vi "updateTimestamp.vi"(8 "error in (no error)":errorcluster, 10 "Timestamp":dbl, 11 "Timestamp in":refnum<class "Timestamp.lvclass">) -> (0 "error out":errorcluster, 3 "Timestamp out":refnum<class "Timestamp.lvclass">)   [LabVIEW 2016, in "RTTimestamp.lvlib" / "Timestamp.lvclass"]
uses:
  Timestamp.lvclass
  Timestamp.lvclass/Timestamp.ctl
  Common_RT_FPGA/IWriteU64FIFO/IWriteU64FIFO.lvclass
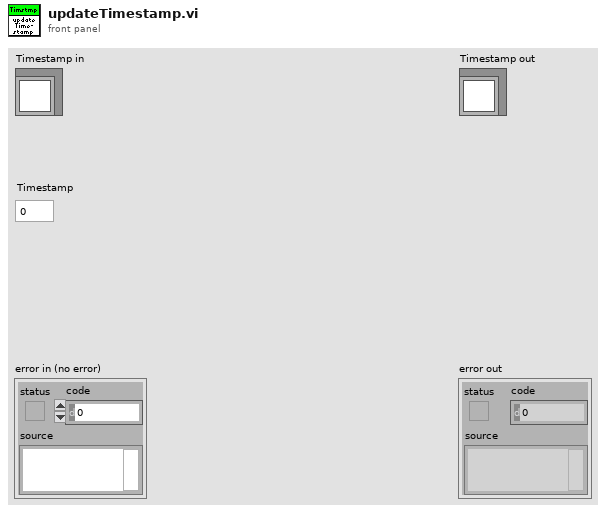
[diagram p1: front panel]
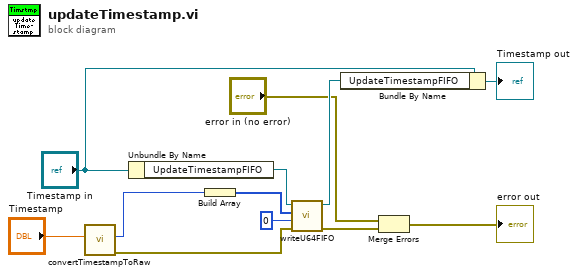
[diagram p0: block diagram]
diagram:
  n1 = call "convertTimestampToRaw.vi"("Timestamp"="Timestamp") -> ("error out"=w2:errorcluster, "Timestamp"=w3:u64)  [unwired: 8 in, 1 out]
  n2 = Unbundle By Name("Timestamp in") -> ("UpdateTimestampFIFO"=w11:refnum<class "IWriteU64FIFO.lvclass">)
  n3 = Build Array(w3) -> (w10:u64[])
  n4 = call-dynamic "writeU64FIFO.vi"("error in (no error)"=w2, "Timeout"=0, "Data"=w10, "IWriteU64FIFO in"=w11) -> ("error out"=w7:errorcluster, "IWriteU64FIFO out"=w8:refnum<class "IWriteU64FIFO.lvclass">)  [unwired: 5 in, 1 out]
  n5 = Bundle By Name(cluster="Timestamp in", "UpdateTimestampFIFO"=w8) -> (→"Timestamp out":refnum<class "Timestamp.lvclass">)
  n6 = Merge Errors("error in (no error)", w7) -> (→"error out":errorcluster)
